vi "Sequence.CreateCase.vi"(7 "Iteration":string, 8 "error in (no error)":errorcluster, 9 "Condition":T1, 10 "Refs":T3, 11 "TaskRef":refnum<k24>) -> (0 "error out":errorcluster)   [LabVIEW 2013, in "Simple Sequence Tools - Editor.lvlib"]
uses:
  Simple Sequence Tools - Editor.lvlib
  Types/Sequence.MainSeqRefs.ctl
  NationalInstruments.VeriStand.RealTimeSequenceDefinitionApi
  Types/Compiled.StepCondition.ctl
  Types/Conditions.OperationTypes.ctl
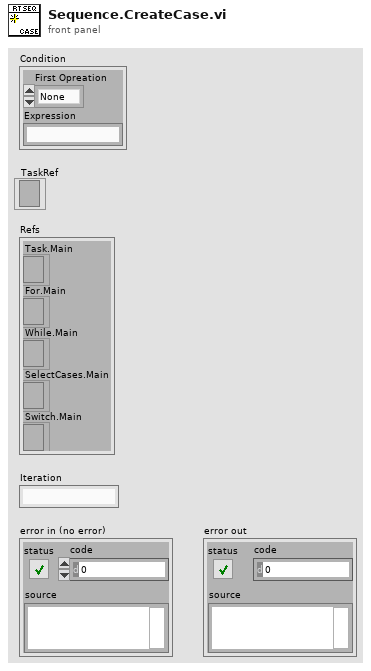
[diagram p1: front panel]
types:
  T1 = typedef "Simple Sequence Tools - Editor.lvlib/Compiled.StepCondition.ctl" = cluster{"First Opreation":T2, "Expression":string}
  T2 = typedef "Simple Sequence Tools - Editor.lvlib/Conditions.OperationTypes.ctl" = enum8{"None", "&&", "||"}
  T3 = typedef "Simple Sequence Tools - Editor.lvlib/Sequence.MainSeqRefs.ctl" = cluster{"Task.Main":refnum<k24>, "For.Main":refnum<k24>, "While.Main":refnum<k24>, "SelectCases.Main":refnum<k24>, "Switch.Main":refnum<k24>}
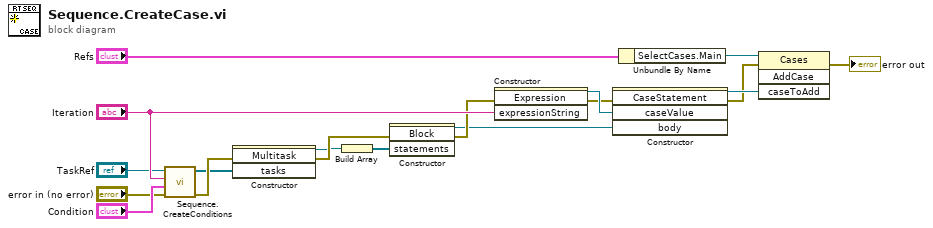
[diagram p0: block diagram]
diagram:
  n1 = call "Sequence.CreateConditions.vi"("error in (no error)"="error in (no error)", "Condition"="Condition", "Iteration"="Iteration", "Task"="TaskRef") -> ("error out"=w14:errorcluster, "Tasks"=w13:refnum<k24>[])  [unwired: 6 in]
  n2 = constructor class="Multitask"(error in=w14, "tasks"=w13) -> (reference out=w10:refnum<k24>, error out=w12:errorcluster)  [unwired: 2 in, 2 out]
  n3 = Build Array(w10) -> (w9:refnum<k24>[])
  n4 = constructor class="Block"(error in=w12, "statements"=w9) -> (reference out=w11:refnum<k24>, error out=w15:errorcluster)  [unwired: 2 in, 2 out]
  n5 = constructor class="Expression"(error in=w15, "expressionString"="Iteration") -> (reference out=w8:refnum<k24>, error out=w4:errorcluster)  [unwired: 2 in, 2 out]
  n6 = constructor class="CaseStatement"(error in=w4, "caseValue"=w8, "body"=w11) -> (reference out=w6:refnum<k24>, error out=w5:errorcluster)  [unwired: 2 in, 3 out]
  n7 = Unbundle By Name("Refs") -> ("SelectCases.Main"=w18:refnum<k24>)
  n8 = invoke class="Cases" method="AddCase"(reference=w18, error in=w5, "caseToAdd"=w6) -> (error out=→"error out":errorcluster)  [unwired: 1 in, 3 out]
